vi "modifier main.vi"() -> ()   [LabVIEW 2013, in "vi mod UI.lvlib"]
doc: "This is the main VI for the configuration editor."
uses:
  vi mod UI.lvlib
  Controls/StateCluster.ctl
  <vilib>/NI/Configuration Framework/Repository/NISE_CEF_Repository.lvclass
  <vilib>/NI/Configuration Framework/Node/NodeRef.ctl
  <vilib>/NI/Configuration Framework/Node/NISE_CEF_Node.lvclass
  <vilib>/NI/Configuration Framework/Node/UserEventRef.ctl
  <vilib>/NI/Configuration Framework/Controls/EventCluster.ctl
  Controls/AddMessage.ctl
  Controls/MoveMessage.ctl
  modification container/modification container.lvclass
  collection/VI modification collection.lvclass
  <vilib>/NI/AMC/Read Termination Message.vi
  <vilib>/NI/AMC/Create Single Message.vi
  <vilib>/NI/AMC/Update Message Routing Info.vi
  <vilib>/NI/AMC/Send Message.vi
  <vilib>/NI/AMC/Globals.vi
  <vilib>/NI/AMC/AMC.lvlib
  <vilib>/NI/Configuration Framework/NISE_CEF_TreeControl.lvlib
panel:
  in  "stop":bool
  in  "View":string(tree)
  # "VI Modifier"
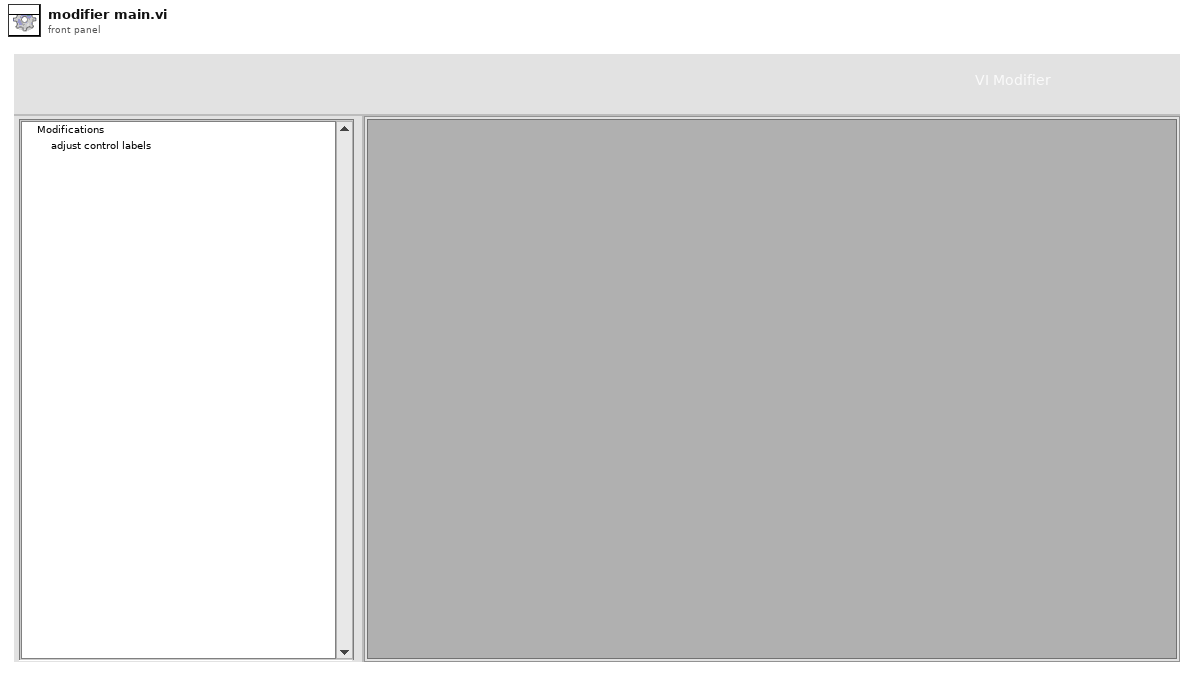
[diagram p1: front panel]
types:
  T1 = typedef "vi mod UI.lvlib/StateCluster.ctl" = cluster{"repository":refnum<class "NISE_CEF_Repository.lvclass">, "root":T2, "unsaved changes":bool, "current path":path, "user event ref":T3, "classes path":path}
  T2 = typedef "NISE_CEF_Node.lvclass/NodeRef.ctl" = refnum<data-value>
  T3 = typedef "NISE_CEF_Node.lvclass/UserEventRef.ctl" = refnum<user-event>
  T4 = typedef "AMC.lvlib/Message Queue.ctl" = refnum<queue>
  T5 = typedef "vi mod UI.lvlib/AddMessage.ctl" = cluster{"node type":string, "to add to":string}
  T6 = typedef "vi mod UI.lvlib/MoveMessage.ctl" = cluster{"node ref":T2, "new parent":T2}
  T7 = typedef "LVPoint32TypeDef.ctl" = cluster{"Horizontal":i32, "Vertical":i32}
  T8 = cluster{"data name":string, "drag data":variant}[]
  T9 = typedef "NISE_CEF_Node.lvclass/NodeMenuOptions.ctl" = cluster{"removable":bool, "movable":bool, "duplicate":bool}
  T10 = typedef "NISE_CEF_TreeControl.lvlib/EventCluster.ctl" = cluster{"command":string, "data":string}
  T11 = typedef "vi mod UI.lvlib/FilePaths.ctl" = cluster{"classes":path}
  T12 = typedef "NISE_CEF_Node.lvclass/Summary.ctl" = cluster{"ID":string, "parent ID":string, "node type":string, "text":string, "additional text":string, "glyph":string, "depth":i32, "glyph overlay":string}
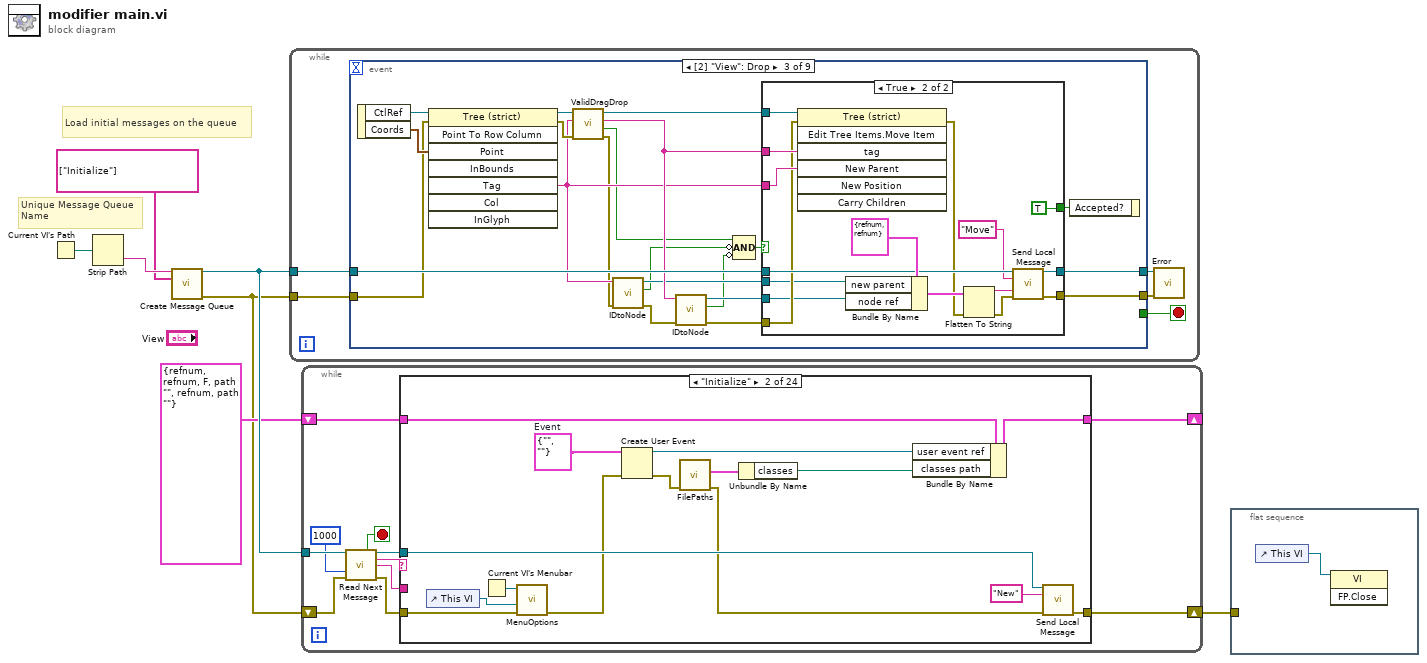
[diagram p0: block diagram]
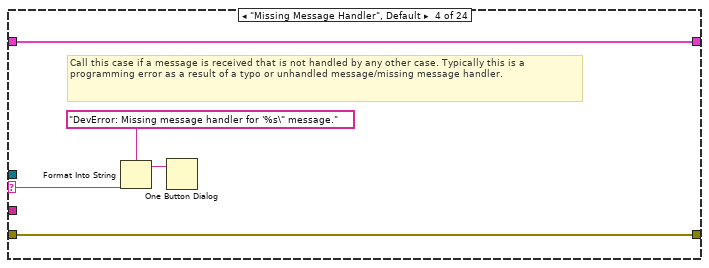
[diagram p4: hidden frame]
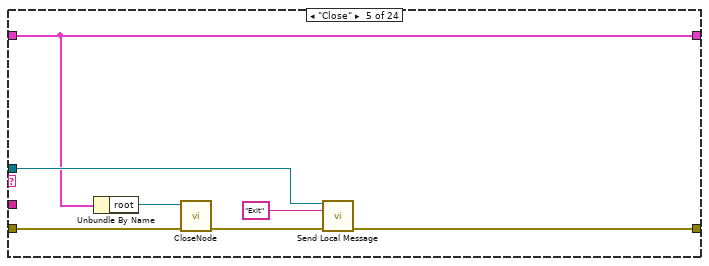
[diagram p5: hidden frame]
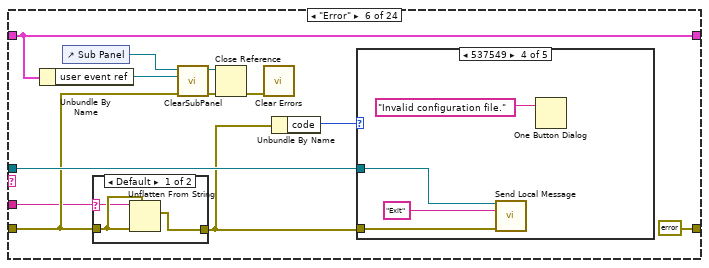
[diagram p6: hidden frame]
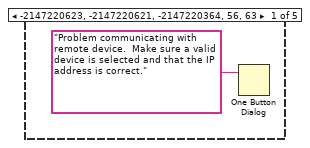
[diagram p8: hidden frame]
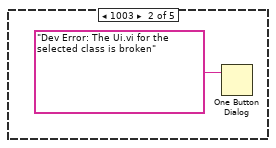
[diagram p9: hidden frame]
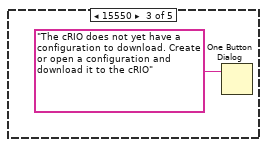
[diagram p10: hidden frame]
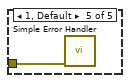
[diagram p11: hidden frame]
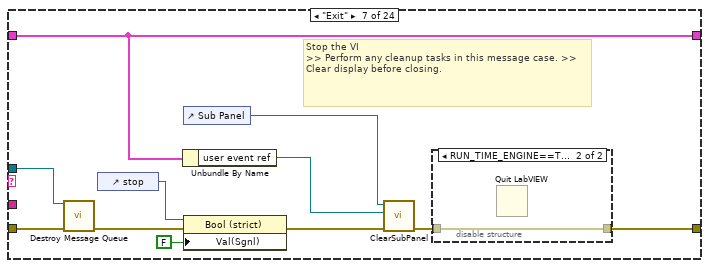
[diagram p12: hidden frame]
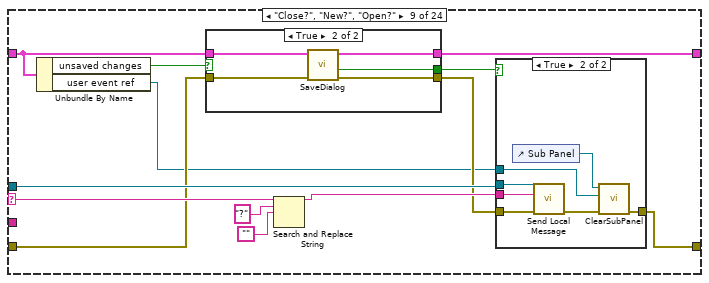
[diagram p15: hidden frame]
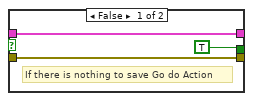
[diagram p16: hidden frame]
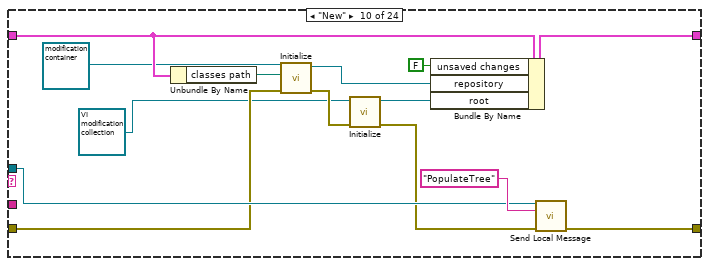
[diagram p18: hidden frame]
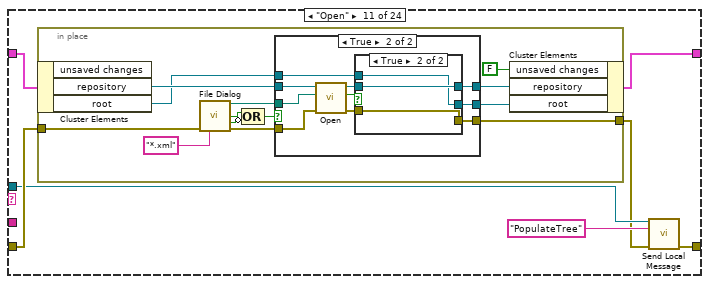
[diagram p19: hidden frame]
diagram:
  # "Unique Message Queue Name"
  # "Load initial messages on the queue"
  n1 = Current VI's Path() -> (path=w6:path)
  n2 = Strip Path(path=w6) -> (name=w7:string)  [unwired: 1 out]
  n3 = call <vilib>:"Create Message Queue.vi"("message queue name"=w7, "initial message names"=string[] ["Initialize"]) -> ("message queue out"=w4:T4, "error out"=w2:errorcluster)  [unwired: 12 in]
  n4 = while "User Interface Event Handler" {
    tunnel: w4 -> [w12]
    tunnel: w2 -> [w8]
    stop <- w11 stop-if-true
    n5 = event shown="[2] \"View\": Drop" {
      selector: _ -> [_ _ _ _ _ _ _ _ _]
      dyn-events: _ -> [_ _ _ _ _ _ _ _ _]
      timeout: _ -> [_ _ _ _ _ _ _ _ _]
      tunnel: w12 -> [w20 w44 w96 w124 w151 w155 w165 w171 w176]
      tunnel: [_ _ _ _ _ _ _ TRUE _] -> w11
      tunnel: [w20 w41 w94 w124 w148 w155 w163 w170 w175] -> w10
      tunnel: [w16 w40 w93 w120 w147 w152 w161 w168 w173] -> w9
      tunnel: w8 -> [w19 w39 w95 w123 w146 w154 w162 w169 w174]
      event "View": Shortcut Menu Activation? {
        n6 = event-data() -> ("CtlRef"=w26:refnum<vi>, "Coords"=w25:T7, "MenuRef"=w22:refnum<k9>)  [unwired: 1 in]
        n7 = invoke class="Tree (strict)" method="Point To Row Column"(reference=w26, error in=w19, "Point"=w25) -> (error out=w18:errorcluster, "Tag"=w24:string)  [unwired: 5 in, 6 out]
        n8 = call <vilib>:"IDtoNode.vi"("error in"=w18, "ID"=w24) -> ("error out"=w14:errorcluster, "invalid Id"=w21:bool, "node ref"=w23:T2)  [unwired: 7 in]
        n9 = case shown="False" w21 {
          tunnel: w23 -> [w31 _]
          tunnel: w22 -> [w30 _]
          tunnel: [w29 _] -> w17
          tunnel: [w28 _] -> w15
          tunnel: w14 -> [w27 w37]
          tunnel: [w27 w37] -> w13
          frame False {
            n10 = in-place {
              in-place-border: w30 -> [w34]
              in-place-border: [w32] -> w29
              n11 = in-place-dvr #1(w31) -> (w36:refnum<class "NISE_CEF_Node.lvclass">, w33:errorcluster)
              n12 = call-dynamic "ShortcutMenu.vi"("error in"=w33, "menu ref in"=w34, "node in"=w36) -> ("error out"=w32:errorcluster, "node out"=w35:refnum<class "NISE_CEF_Node.lvclass">)  [unwired: 6 in, 1 out]
              n13 = in-place-dvr #1(w35) -> (w28:errorcluster)  [unwired: 1 out]
            }
          }
          frame True {
          }
        }
        n14 = Merge Errors(w15, w17, w13) -> (w16:errorcluster)
        n15 = event-data() -> ()  [unwired: 2 in, 1 out]
      }
      event "View": Shortcut Menu Selection (User) {
        n16 = event-data() -> ("ItemPath"=w43:string, "CtlRef"=w47:refnum<vi>, "Coords"=w48:T7)  [unwired: 1 in]
        n17 = invoke class="Tree (strict)" method="Point To Row Column"(reference=w47, error in=w39, "Point"=w48) -> (error out=w38:errorcluster, "Tag"=w42:string)  [unwired: 5 in, 6 out]
        n18 = Match Pattern(string=w43, regular expression=":") -> (before substring=w46:string, after substring=w45:string)  [unwired: 1 in, 2 out]
        n19 = case shown="Default" w46 {
          selector: w46 -> [w50 _ _ _]
          tunnel: w45 -> [_ _ _ w75]
          tunnel: w44 -> [w57 w64 w70 w77]
          tunnel: w42 -> [w52 w62 w68 w76]
          tunnel: [w54 w61 w67 w73] -> w41
          tunnel: [w55 w60 w65 w71] -> w40
          tunnel: w38 -> [w56 w59 w66 w72]
          frame Default {
            n20 = Concatenate Strings(w50, ":" ("string"), w52) -> (w53:string)
            n21 = call <vilib>:"Send Local Message.vi"("message queue in"=w57, "message name"="CustomMenuAction" ("Message Name"), "message value"=w53, "error in"=w56) -> ("message queue out"=w54:T4, "error out"=w55:errorcluster)  [unwired: 9 in, 1 out]
          }
          frame "Remove" {
            n22 = call <vilib>:"Send Local Message.vi"("message queue in"=w64, "message name"="RemoveNode" ("Message Name"), "message value"=w62, "error in"=w59) -> ("message queue out"=w61:T4, "error out"=w60:errorcluster)  [unwired: 9 in, 1 out]
          }
          frame "Duplicate" {
            n23 = call <vilib>:"Send Local Message.vi"("message queue in"=w70, "message name"="Duplicate" ("Message Name"), "message value"=w68, "error in"=w66) -> ("message queue out"=w67:T4, "error out"=w65:errorcluster)  [unwired: 9 in, 1 out]
          }
          frame "Add" {
            n24 = Bundle By Name(cluster=T5 {"node type"="", "to add to"=""} ("input cluster"), "node type"=w75, "to add to"=w76) -> (w78:T5)
            n25 = Flatten To String(anything=w78) -> (data string=w79:string)  [unwired: 3 in, 2 out]
            n26 = call <vilib>:"Send Local Message.vi"("message queue in"=w77, "message name"="AddNode" ("Message Name"), "message value"=w79, "error in"=w72) -> ("message queue out"=w73:T4, "error out"=w71:errorcluster)  [unwired: 9 in, 1 out]
          }
        }
      }
      event "View": Drop {
        n27 = event-data() -> ("CtlRef"=w99:refnum<vi>, "Coords"=w98:T7)  [unwired: 1 in]
        n28 = invoke class="Tree (strict)" method="Point To Row Column"(reference=w99, error in=w95, "Point"=w98) -> (reference out=w97:refnum<vi>, error out=w92:errorcluster, "Tag"=w89:string)  [unwired: 5 in, 5 out]
        n29 = call <vilib>:"ValidDragDrop.vi"("error in"=w92, "drag over"=w89, "tree ref in"=w97) -> ("error out"=w84:errorcluster, "accepted"=w87:bool, "drag"=w91:string, "tree ref out"=w101:refnum<vi>)  [unwired: 5 in]
        n30 = call <vilib>:"IDtoNode.vi"("error in"=w84, "ID"=w89) -> ("error out"=w85:errorcluster, "invalid Id"=w82:bool, "node ref"=w88:T2)  [unwired: 7 in]
        n31 = call <vilib>:"IDtoNode.vi"("error in"=w85, "ID"=w91) -> ("error out"=w83:errorcluster, "invalid Id"=w81:bool, "node ref"=w90:T2)  [unwired: 7 in]
        n32 = Compound Arithmetic op=AND(w87, invert w82, invert w81) -> (w86:bool)
        n33 = case shown="True" w86 {
          tunnel: w91 -> [_ w117]
          tunnel: w101 -> [_ w119]
          tunnel: [_ TRUE] -> w100
          tunnel: w89 -> [_ w115]
          tunnel: w96 -> [w103 w114]
          tunnel: [w103 w110] -> w94
          tunnel: [w102 w109] -> w93
          tunnel: w90 -> [_ w105]
          tunnel: w88 -> [_ w104]
          tunnel: w83 -> [w102 w106]
          frame False {
          }
          frame True {
            n34 = invoke class="Tree (strict)" method="Edit Tree Items.Move Item"(reference=w119, error in=w106, "tag"=w117, "New Parent"=w115) -> (error out=w107:errorcluster)  [unwired: 3 in, 6 out]
            n35 = Bundle By Name(cluster=T6 {"node ref"=refnum, "new parent"=refnum} ("Cluster"), "new parent"=w104, "node ref"=w105) -> (w113:T6)
            n36 = Flatten To String(anything=w113, error in (no error)=w107) -> (data string=w112:string, error out=w108:errorcluster)  [unwired: 2 in, 1 out]
            n37 = call <vilib>:"Send Local Message.vi"("message queue in"=w114, "message name"="Move", "message value"=w112, "error in"=w108) -> ("message queue out"=w110:T4, "error out"=w109:errorcluster)  [unwired: 9 in, 1 out]
          }
        }
        n38 = event-data("Accepted?"=w100) -> ()  [unwired: 1 in, 1 out]
      }
      event "View": Drag Starting? {
        n39 = event-data() -> ("Data"=w130:T8, "CtlRef"=w132:refnum<vi>, "Coords"=w131:T7)  [unwired: 1 in]
        n40 = invoke class="Tree (strict)" method="Point To Row Column"(reference=w132, error in=w123, "Point"=w131) -> (error out=w122:errorcluster, "Tag"=w129:string)  [unwired: 5 in, 6 out]
        n41 = call <vilib>:"IDtoNode.vi"("error in"=w122, "ID"=w129) -> ("error out"=w121:errorcluster, "invalid Id"=w128:bool, "node ref"=w127:T2)  [unwired: 7 in]
        n42 = case shown="False" w128 {
          tunnel: w127 -> [w138 _]
          tunnel: [w135 TRUE ("Removable")] -> w125
          tunnel: w121 -> [w134 w144]
          tunnel: [w133 w144] -> w120
          frame False {
            n43 = in-place {
              in-place-border: [w141] -> w137
              in-place-border: w134 -> [w140]
              in-place-border: [w139] -> w133
              n44 = in-place-dvr #2(w138) -> (w143:refnum<class "NISE_CEF_Node.lvclass">)  [unwired: 1 out]
              n45 = call-dynamic "EditOptions.vi"("error in"=w140, "node in"=w143) -> ("error out"=w139:errorcluster, "edit options"=w141:T9, "node out"=w142:refnum<class "NISE_CEF_Node.lvclass">)  [unwired: 6 in, 1 out]
              n46 = in-place-dvr #2(w142) -> ()  [unwired: 2 out]
            }
            n47 = Unbundle By Name(w137) -> ("movable"=w136:bool)
            n48 = Not(x=w136) -> (.not. x?=w135:bool)
          }
          frame True {
          }
        }
        n49 = event-data("Data"=w130, "Drag Mode"=enum32{"copy or move", "copy only", "move only"}."move only", "Discard?"=w125) -> ()  [unwired: 1 in, 1 out]
      }
      event "View": Value Change {
        n50 = event-data() -> ("NewVal"=w149:string)  [unwired: 1 in]
        n51 = call <vilib>:"Send Local Message.vi"("message queue in"=w151, "message name"="ActivateNode" ("Message Name"), "message value"=w149, "error in"=w146) -> ("message queue out"=w148:T4, "error out"=w147:errorcluster)  [unwired: 9 in, 1 out]
      }
      event "View": event type 3.0.xa000003a {
        n52 = event-data() -> ("CtlRef"=w160:refnum<vi>, "Coords"=w157:T7)  [unwired: 1 in]
        n53 = invoke class="Tree (strict)" method="Point To Row Column"(reference=w160, error in=w154, "Point"=w157) -> (reference out=w159:refnum<vi>, error out=w153:errorcluster, "Tag"=w158:string)  [unwired: 5 in, 5 out]
        n54 = call <vilib>:"ValidDragDrop.vi"("error in"=w153, "drag over"=w158, "tree ref in"=w159) -> ("error out"=w152:errorcluster, "accepted"=w156:bool)  [unwired: 5 in, 2 out]
        n55 = event-data("Accepted?"=w156) -> ()  [unwired: 1 in, 1 out]
      }
      event Panel Close? {
        # "Intercepts the upper right close panel operation to allow a smooth shutdown as opposed to immediately killing the app."
        n56 = event-data() -> ()  [unwired: 1 in, 1 out]
        n57 = call <vilib>:"Send Local Message.vi"("message queue in"=w165, "message name"="Close?", "error in"=w162) -> ("message queue out"=w163:T4, "error out"=w161:errorcluster)  [unwired: 10 in, 1 out]
        n58 = event-data("Discard?"=TRUE) -> ()  [unwired: 1 in, 1 out]
      }
      event "stop": Value Change {
        n59 = event-data() -> ()  [unwired: 1 in, 1 out]
        n60 = call <vilib>:"Send Local Message.vi"("message queue in"=w171, "message name"="Close", "error in"=w169) -> ("message queue out"=w170:T4, "error out"=w168:errorcluster)  [unwired: 10 in, 1 out]
      }
      event Menu Selection (User) {
        # "#USERCFG It is needed to add a Case for Every item on the menu"
        n61 = event-data() -> ("ItemPath"=w177:string)  [unwired: 1 in]
        n62 = case shown="Default" w177 {
          tunnel: w176 -> [w179 w185 w190 w195 w200 w205 w214]
          tunnel: [w179 w181 w186 w191 w196 w201 w211] -> w175
          tunnel: w174 -> [w178 w183 w188 w193 w198 w203 w210]
          tunnel: [w178 w182 w187 w192 w197 w202 w208] -> w173
          frame Default {
            n63 = One Button Dialog(message="Unknown Menu Option") -> ()  [unwired: 1 in, 1 out]
          }
          frame "_File:_New" {
            n64 = call <vilib>:"Send Local Message.vi"("message queue in"=w185, "message name"="New?" ("Message Name"), "error in"=w183) -> ("message queue out"=w181:T4, "error out"=w182:errorcluster)  [unwired: 10 in, 1 out]
          }
          frame "_File:_Open" {
            n65 = call <vilib>:"Send Local Message.vi"("message queue in"=w190, "message name"="Open?" ("Message Name"), "error in"=w188) -> ("message queue out"=w186:T4, "error out"=w187:errorcluster)  [unwired: 10 in, 1 out]
          }
          frame "_File:_Save" {
            n66 = call <vilib>:"Send Local Message.vi"("message queue in"=w195, "message name"="Save" ("Message Name"), "error in"=w193) -> ("message queue out"=w191:T4, "error out"=w192:errorcluster)  [unwired: 10 in, 1 out]
          }
          frame "_File:Save As..." {
            n67 = call <vilib>:"Send Local Message.vi"("message queue in"=w200, "message name"="SaveAs" ("Message Name"), "error in"=w198) -> ("message queue out"=w196:T4, "error out"=w197:errorcluster)  [unwired: 10 in, 1 out]
          }
          frame "_File:_Exit" {
            n68 = call <vilib>:"Send Local Message.vi"("message queue in"=w205, "message name"="Close?" ("Message Name"), "error in"=w203) -> ("message queue out"=w201:T4, "error out"=w202:errorcluster)  [unwired: 10 in, 1 out]
          }
          frame "_Tools:Multiple Parameter Editor" {
            n69 = call <vilib>:"Send Local Message.vi"("message queue in"=w214, "message name"="CleansubPanel", "error in"=w210) -> ("message queue out"=w213:T4, "error out"=w209:errorcluster)  [unwired: 10 in, 1 out]
            n70 = call <vilib>:"Send Local Message.vi"("message queue in"=w213, "message name"="Custom View" ("Message Name"), "message value"="Multiple Variable Editor" ("Message Name"), "error in"=w209) -> ("message queue out"=w211:T4, "error out"=w208:errorcluster)  [unwired: 9 in, 1 out]
          }
        }
      }
    }
    n71 = call "Error.vi"("error in (no error)"=w9, "message queue in"=w10) -> ()  [unwired: 9 in, 1 out]
  }
  n72 = while "Message Processor" {
    shift-right: [w221] -> w1
    shift-left: w2 -> [w220]
    tunnel: w4 -> [w219]
    shift-right: [w217] -> _
    shift-left: T1 {"repository"=refnum, "root"=refnum, "unsaved changes"=FALSE, "current path"=path "", "user event ref"=refnum, "classes path"=path ""} -> [w216]
    stop <- w225 stop-if-true
    n73 = call <vilib>:"Read Next Message.vi"("message queue in"=w219, "timeout (1 ms)"=1000, "error in"=w220) -> ("exit process?"=w225:bool, "message queue out"=w215:T4, "message name"=w224:string, "message value"=w223:string, "error out"=w222:errorcluster)  [unwired: 5 in, 3 out]
    n74 = case shown="\"Initialize\"" w224 {
      selector: w224 -> [_ _ _ w246 _ _ _ _ w304 _ _ _ _ _ _ _ _ w487 _ _ _ _ _ _]
      tunnel: w223 -> [_ _ _ _ _ w257 _ _ _ _ _ _ _ w416 _ w455 w468 w485 w516 w539 _ _ w575 w597]
      tunnel: w222 -> [w227 w242 w244 w249 w251 w260 w291 w295 w297 w327 w343 w382 w408 w423 w436 w444 w467 w490 w518 w538 w555 w565 w574 w595]
      tunnel: [w227 w238 w244 w249 w255 errorcluster {"status"=FALSE, "code"=0, "source"=""} ("error out") w284 w295 w308 w337 w339 w386 w410 w420 w436 w447 w471 w493 w522 w535 w549 w560 w571 w590] -> w221
      tunnel: [w226 w233 w243 w245 w253 w265 w283 w294 w299 w335 w344 w389 w409 w417 w435 w438 w465 w494 w520 w533 w559 w564 w569 w586] -> w217
      tunnel: w216 -> [w226 w234 w243 w245 w253 w265 w283 w294 w300 w331 w345 w384 w407 w418 w435 w442 w472 w494 w521 w540 w559 w564 w569 w598]
      tunnel: w215 -> [_ w237 _ _ w254 w268 w290 _ w307 w336 w341 w385 _ w419 _ _ _ w488 _ _ _ _ w570 w589]
      frame "------------Generic Operations------------" {
        # "Dummy case to add a seperation in the Case Structure menu"
      }
      frame "Initialize" {
        w229 = T10 {"command"="", "data"=""}  # Event
        n75 = control-ref of="This VI"() -> (w241:refnum<vi>)
        n76 = Current VI's Menubar() -> (w240:refnum<k9>)
        n77 = call "MenuOptions.vi"("error in"=w242, "VI ref"=w241, "menu ref in"=w240) -> ("error out"=w232:errorcluster)  [unwired: 7 in, 1 out]
        n78 = Create User Event(user event datatype=w229, error in=w232) -> (user event=w228:refnum<user-event>, error out=w231:errorcluster)
        n79 = call "FilePaths.vi"("error in"=w231) -> ("error out"=w236:errorcluster, "paths"=w235:T11)  [unwired: 9 in]
        n80 = Unbundle By Name(w235) -> ("classes"=w230:path)
        n81 = Bundle By Name(cluster=w234, "user event ref"=w228, "classes path"=w230) -> (w233:T1)
        n82 = call <vilib>:"Send Local Message.vi"("message queue in"=w237, "message name"="New" ("Message Name"), "error in"=w236) -> ("error out"=w238:errorcluster)  [unwired: 10 in, 2 out]
      }
      frame "", "Idle" {
      }
      frame "Missing Message Handler", Default {
        # "Call this case if a message is received that is not handled by any other case. Typically this is a programming error as a result of a typo or unhandled message/missing message handler."
        n83 = Format Into String(format string="DevError: Missing message handler for '%s\" message." ("message"), w246) -> (resulting string=w248:string)  [unwired: 2 in, 1 out]
        n84 = One Button Dialog(message=w248) -> ()  [unwired: 2 out]
      }
      frame "Close" {
        n85 = Unbundle By Name(w253) -> ("root"=w252:T2)
        n86 = call <vilib>:"CloseNode.vi"("error in"=w251, "node ref"=w252) -> ("error out"=w250:errorcluster)  [unwired: 9 in]
        n87 = call <vilib>:"Send Local Message.vi"("message queue in"=w254, "message name"="Exit", "error in"=w250) -> ("error out"=w255:errorcluster)  [unwired: 10 in, 2 out]
      }
      frame "Error" {
        n88 = Unbundle By Name(w265) -> ("user event ref"=w263:T3)
        n89 = control-ref of="Sub Panel"() -> (w264:refnum<vi>)
        n90 = case shown="Default" w257 {
          selector: w257 -> [w270 _]
          tunnel: w260 -> [w271 w272]
          tunnel: [w269 w272] -> w259
          frame Default {
            n91 = Unflatten From String(type=w271, binary string=w270, error in (no error)=w271) -> (value=w269:errorcluster)  [unwired: 2 in, 2 out]
          }
          frame "" {
          }
        }
        n92 = call <vilib>:"ClearSubPanel.vi"("error in"=w260, "user event ref"=w263, "sub panel ref in"=w264) -> ("error out"=w262:errorcluster, "sub panel ref out"=w261:refnum<vi>)  [unwired: 7 in]
        n93 = Close Reference(reference=w261, error in (no error)=w262) -> (error out=w258:errorcluster)
        n94 = call <vilib>:"Clear Errors.vi"("error in (no error)"=w258) -> ()  [unwired: 6 in, 1 out]
        n95 = Unbundle By Name(w259) -> ("code"=w266:i32)
        n96 = case shown="537549" w266 {
          tunnel: w268 -> [_ _ _ w278 _]
          tunnel: w259 -> [_ _ _ w277 w280]
          frame -2147220623, -2147220621, -2147220364, 56, 63 {
            n97 = One Button Dialog(message="Problem communicating with remote device.  Make sure a valid device is selected and that the IP address is correct.") -> ()  [unwired: 1 in, 1 out]
          }
          frame 1003 {
            n98 = One Button Dialog(message="Dev Error: The Ui.vi for the selected class is broken") -> ()  [unwired: 1 in, 1 out]
          }
          frame 15550 {
            n99 = One Button Dialog(message="The cRIO does not yet have a configuration to download. Create or open a configuration and download it to the cRIO") -> ()  [unwired: 1 in, 1 out]
          }
          frame 537549 {
            n100 = call <vilib>:"Send Local Message.vi"("message queue in"=w278, "message name"="Exit", "error in"=w277) -> ()  [unwired: 10 in, 3 out]
            n101 = One Button Dialog(message="Invalid configuration file.") -> ()  [unwired: 1 in, 1 out]
          }
          frame 1, Default {
            n102 = call <vilib>:"Simple Error Handler.vi"("error in (no error)"=w280) -> ()  [unwired: 1 in, 8 out]
          }
        }
      }
      frame "Exit" {
        # "Stop the VI                                                                             >> Perform any cleanup tasks in this message case. >> Clear display before closing."
        n103 = call <vilib>:"Destroy Message Queue.vi"("message queue in"=w290, "error in"=w291) -> ("error out"=w288:errorcluster)  [unwired: 11 in, 2 out]
        n104 = control-ref of="stop"() -> (w281:refnum<vi>)
        n105 = Unbundle By Name(w283) -> ("user event ref"=w282:T3)
        n106 = control-ref of="Sub Panel"() -> (w287:refnum<vi>)
        n107 = property class="Bool (strict)"(reference=w281, error in=w288, "Val(Sgnl)"=FALSE ("Exit")) -> (error out=w286:errorcluster)  [unwired: 1 out]
        n108 = call <vilib>:"ClearSubPanel.vi"("error in"=w286, "user event ref"=w282, "sub panel ref in"=w287) -> ("error out"=w285:errorcluster)  [unwired: 7 in, 1 out]
        n109 = disable-structure shown="RUN_TIME_ENGINE==True" {
          disable-tunnel: [w292 w293] -> w284
          disable-tunnel: w285 -> [w292 w293]
          frame condition #0 (active) {
          }
          frame condition #1 {
            n110 = Quit LabVIEW() -> ()  [unwired: 1 in]
          }
        }
      }
      frame "------------Menu Operations--------------" {
        # "Dummy case to add a seperation in the Case Structure menu"
      }
      frame "Close?", "New?", "Open?" {
        n111 = Unbundle By Name(w300) -> ("unsaved changes"=w302:bool, "user event ref"=w296:T3)
        n112 = case shown="True" w302 {
          tunnel: [TRUE ("SaveFlag") w316] -> w301
          tunnel: w300 -> [w310 w315]
          tunnel: [w310 w314] -> w299
          tunnel: w297 -> [w309 w313]
          tunnel: [w309 w312] -> w298
          frame False {
            # "If there is nothing to save Go do Action"
          }
          frame True {
            n113 = call "SaveDialog.vi"("error in"=w313, "state in"=w315) -> ("error out"=w312:errorcluster, "new"=w316:bool, "state out"=w314:T1)  [unwired: 7 in]
          }
        }
        n114 = Search and Replace String(input string=w304, search string="?", replace string="") -> (result string=w303:string)  [unwired: 5 in, 3 out]
        n115 = case shown="True" w301 {
          tunnel: w298 -> [w317 w324]
          tunnel: [w317 w320] -> w308
          tunnel: w307 -> [_ w323]
          tunnel: w303 -> [_ w322]
          tunnel: w296 -> [_ w319]
          frame False {
          }
          frame True {
            n116 = control-ref of="Sub Panel"() -> (w318:refnum<vi>)
            n117 = call <vilib>:"Send Local Message.vi"("message queue in"=w323, "message name"=w322, "error in"=w324) -> ("error out"=w321:errorcluster)  [unwired: 10 in, 2 out]
            n118 = call <vilib>:"ClearSubPanel.vi"("error in"=w321, "user event ref"=w319, "sub panel ref in"=w318) -> ("error out"=w320:errorcluster)  [unwired: 7 in, 1 out]
          }
        }
      }
      frame "New" {
        n119 = Unbundle By Name(w331) -> ("classes path"=w330:path)
        n120 = call-dynamic "Initialize.vi"("error in"=w327, "path"=w330, "repository in"=refnum<class "modification container.lvclass"> refnum ("modification container.lvclass")) -> ("error out"=w329:errorcluster, "repository out"=w332:refnum<class "modification container.lvclass">)  [unwired: 7 in]
        n121 = call-dynamic "Initialize.vi"("error in"=w329, "node in"=refnum<class "VI modification collection.lvclass"> refnum ("VI modification collection.lvclass")) -> ("error out"=w328:errorcluster, "data value reference"=w333:T2)  [unwired: 7 in, 1 out]
        n122 = Bundle By Name(cluster=w331, "unsaved changes"=FALSE ("SaveFlag"), "repository"=w332, "root"=w333) -> (w335:T1)
        n123 = call <vilib>:"Send Local Message.vi"("message queue in"=w336, "message name"="PopulateTree", "error in"=w328) -> ("error out"=w337:errorcluster)  [unwired: 10 in, 2 out]
      }
      frame "Open" {
        n124 = in-place {
          in-place-border: w343 -> [w351]
          in-place-border: [w355] -> w340
          n125 = in-place-cluster #3(w345) -> ("repository"=w358:refnum<class "NISE_CEF_Repository.lvclass">, "root"=w349:T2)  [unwired: 1 out]
          n126 = call "File Dialog"("error in"=w351, "pattern (all files)"="*.xml") -> ("selected path"=w352:path, "exists"=w348:bool, "cancelled"=w347:bool, "error out"=w350:errorcluster)  [unwired: 10 in]
          n127 = Compound Arithmetic op=OR(w348, invert w347) -> (w346:bool)
          n128 = case shown="True" w346 {
            tunnel: w358 -> [w359 w371]
            tunnel: [w359 w369] -> w356
            tunnel: [w360 w367] -> w355
            tunnel: [w361 w366] -> w354
            tunnel: w352 -> [_ w364]
            tunnel: w350 -> [w360 w363]
            tunnel: w349 -> [w361 w362]
            frame False {
            }
            frame True {
              n129 = call-dynamic "Open.vi"("error in"=w363, "file path"=w364, "repository in"=w371) -> ("error out"=w368:errorcluster, "invalid?"=w365:bool, "repository out"=w370:refnum<class "NISE_CEF_Repository.lvclass">)  [unwired: 6 in]
              n130 = case shown="True" w365 {
                tunnel: w370 -> [w376 w379]
                tunnel: [w375 w379] -> w369
                tunnel: w368 -> [w374 w378]
                tunnel: [w373 w378] -> w367
                tunnel: [w372 w377] -> w366
                tunnel: w362 -> [_ w377]
                frame False {
                  n131 = call-dynamic "WriteTree.vi"("error in"=w374, "repository in"=w376) -> ("error out"=w373:errorcluster, "root"=w372:T2, "repository out"=w375:refnum<class "NISE_CEF_Repository.lvclass">)  [unwired: 7 in]
                }
                frame True {
                }
              }
            }
          }
          n132 = in-place-cluster #3("unsaved changes"=FALSE ("SaveFlag"), "repository"=w356, "root"=w354) -> (w344:T1)
        }
        n133 = call <vilib>:"Send Local Message.vi"("message queue in"=w341, "message name"="PopulateTree", "error in"=w340) -> ("error out"=w339:errorcluster)  [unwired: 10 in, 2 out]
      }
      frame "Save" {
        n134 = in-place {
          in-place-border: w382 -> [w393]
          in-place-border: [w392] -> w381
          in-place-border: [w390] -> w380
          n135 = in-place-cluster #4(w384) -> ("current path"=w391:path, "root"=w394:T2, "repository"=w396:refnum<class "NISE_CEF_Repository.lvclass">)
          n136 = Empty String/Path?(string/path=w391) -> (empty?=w390:bool)
          n137 = call-dynamic "ReadTree.vi"("error in"=w393, "root"=w394, "repository in"=w396) -> ("error out"=w392:errorcluster, "repository out"=w395:refnum<class "NISE_CEF_Repository.lvclass">)  [unwired: 7 in]
          n138 = in-place-cluster #4("current path"=w391, "root"=w394, "repository"=w395) -> (w383:T1)
        }
        n139 = case shown="True" w380 {
          tunnel: w383 -> [w400 w402]
          tunnel: [w399 w401] -> w389
          tunnel: [w398 w403] -> w387
          tunnel: w381 -> [w397 w404]
          frame False {
            n140 = call "Save.vi"("error in"=w397, "state in"=w400) -> ("error out"=w398:errorcluster, "state out"=w399:T1)  [unwired: 8 in]
          }
          frame True {
            # "Empty path use Dialog"
            n141 = call "SaveAs.vi"("error in"=w404, "state in"=w402) -> ("error out"=w403:errorcluster, "state out"=w401:T1)  [unwired: 7 in, 1 out]
          }
        }
        n142 = call <vilib>:"Send Local Message.vi"("message queue in"=w385, "message name"="PopulateTree", "error in"=w387) -> ("error out"=w386:errorcluster)  [unwired: 10 in, 2 out]
      }
      frame "SaveAs" {
        n143 = in-place {
          in-place-border: w408 -> [w412]
          in-place-border: [w411] -> w406
          n144 = in-place-cluster #5(w407) -> ("root"=w413:T2, "repository"=w415:refnum<class "NISE_CEF_Repository.lvclass">)
          n145 = call-dynamic "ReadTree.vi"("error in"=w412, "root"=w413, "repository in"=w415) -> ("error out"=w411:errorcluster, "repository out"=w414:refnum<class "NISE_CEF_Repository.lvclass">)  [unwired: 7 in]
          n146 = in-place-cluster #5("root"=w413, "repository"=w414) -> (w405:T1)
        }
        n147 = call "SaveAs.vi"("error in"=w406, "state in"=w405) -> ("error out"=w410:errorcluster, "state out"=w409:T1)  [unwired: 7 in, 1 out]
      }
      frame "Custom View" {
        n148 = in-place {
          in-place-border: w423 -> [w434]
          in-place-border: [w433] -> w421
          in-place-border: w416 -> [w424]
          n149 = in-place-cluster #6(w418) -> ("repository"=w428:refnum<class "NISE_CEF_Repository.lvclass">, "root"=w427:T2)
          n150 = call-dynamic "ReadTree.vi"("error in"=w434, "root"=w427, "repository in"=w428) -> ("error out"=w431:errorcluster, "repository out"=w430:refnum<class "NISE_CEF_Repository.lvclass">)  [unwired: 7 in]
          n151 = call-dynamic "CustomView.vi"("error in"=w431, "view name"=w424, "repository in"=w430) -> ("error out"=w432:errorcluster, "repository out"=w429:refnum<class "NISE_CEF_Repository.lvclass">)  [unwired: 7 in]
          n152 = call-dynamic "WriteTree.vi"("error in"=w432, "repository in"=w429) -> ("error out"=w433:errorcluster, "root"=w425:T2, "repository out"=w426:refnum<class "NISE_CEF_Repository.lvclass">)  [unwired: 7 in]
          n153 = in-place-cluster #6("repository"=w426, "root"=w425) -> (w417:T1)
        }
        n154 = call <vilib>:"Send Local Message.vi"("message queue in"=w419, "message name"="PopulateTree", "error in"=w421) -> ("error out"=w420:errorcluster)  [unwired: 10 in, 2 out]
      }
      frame "-------TreeControl Operations-----------" {
        # "Dummy case to add a seperation in the Case Structure menu"
      }
      frame "AddNode" {
        n155 = Unflatten From String(type=T5 {"node type"="", "to add to"=""} ("input cluster"), binary string=w455) -> (value=w453:T5)  [unwired: 3 in, 2 out]
        n156 = Unbundle By Name(w453) -> ("to add to"=w450:string, "node type"=w440:string)
        n157 = in-place {
          in-place-border: w444 -> [w461]
          in-place-border: [w460] -> w443
          in-place-border: w440 -> [w459]
          in-place-border: [w458] -> w439
          n158 = in-place-cluster #7(w442) -> ("repository"=w463:refnum<class "NISE_CEF_Repository.lvclass">)
          n159 = call-dynamic "GetClassPath.vi"("error in"=w461, "class name"=w459, "Repository in"=w463) -> ("error out"=w460:errorcluster, "class path"=w458:path, "Repository out"=w462:refnum<class "NISE_CEF_Repository.lvclass">)  [unwired: 6 in]
          n160 = in-place-cluster #7("repository"=w462) -> (w441:T1)
        }
        n161 = control-ref of="View"() -> (w445:refnum<vi>)
        n162 = call <vilib>:"Get LV Class Default Value.vi"("error in (no error)"=w443, "class path"=w439) -> ("error out"=w456:errorcluster, "object"=w457:refnum<class>)  [unwired: 8 in]
        n163 = To More Specific Class(target class=refnum<class "NISE_CEF_Node.lvclass"> refnum ("Node.lvclass"), reference=w457, error in=w456) -> (specific class reference=w452:refnum<class "NISE_CEF_Node.lvclass">, error out=w449:errorcluster)
        n164 = Bundle By Name(cluster=w441, "unsaved changes"=TRUE) -> (w438:T1)
        n165 = call <vilib>:"AddNode.vi"("error in"=w449, "node in"=w452, "parent node ID"=w450) -> ("error out"=w448:errorcluster, "summary"=w446:T12[])  [unwired: 7 in]
        n166 = call <vilib>:"PopulateTreeSumary.vi"("error in"=w448, "array"=w446, "tree ref in"=w445) -> ("error out"=w447:errorcluster)  [unwired: 8 in]
      }
      frame "Duplicate" {
        n167 = call <vilib>:"IDtoNode.vi"("error in"=w467, "ID"=w468) -> ("error out"=w469:errorcluster, "invalid Id"=w466:bool, "node ref"=w470:T2)  [unwired: 7 in]
        n168 = case shown="False" w466 {
          tunnel: [w481 w482] -> w471
          tunnel: w470 -> [w479 _]
          tunnel: w469 -> [w476 w482]
          frame False {
            n169 = call <vilib>:"DuplicateNode.vi"("same parent?"=TRUE ("s"), "error in"=w476, "node ref in"=w479) -> ("error out"=w477:errorcluster, "new node ref"=w478:T2)  [unwired: 7 in]
            n170 = call <vilib>:"Summary.vi"("error in"=w477, "node self ref"=w478) -> ("error out"=w474:errorcluster, "summary"=w473:T12[])  [unwired: 8 in]
            n171 = control-ref of="View"() -> (w480:refnum<vi>)
            n172 = call <vilib>:"PopulateTreeSumary.vi"("error in"=w474, "array"=w473, "tree ref in"=w480) -> ("error out"=w481:errorcluster)  [unwired: 8 in]
          }
          frame True {
          }
        }
        n173 = Bundle By Name(cluster=w472, "unsaved changes"=TRUE) -> (w465:T1)
      }
      frame "CustomMenuAction" {
        n174 = Match Pattern(string=w485, regular expression=":") -> (before substring=w484:string, after substring=w483:string)  [unwired: 1 in, 2 out]
        n175 = call <vilib>:"IDtoNode.vi"("error in"=w490, "ID"=w483) -> ("error out"=w491:errorcluster, "invalid Id"=w489:bool, "node ref"=w492:T2)  [unwired: 7 in]
        n176 = case shown="False" w489 {
          tunnel: [w497 w513] -> w493
          tunnel: w492 -> [w501 _]
          tunnel: w491 -> [w498 w513]
          tunnel: w488 -> [w500 _]
          tunnel: w487 -> [_ _]
          tunnel: w484 -> [w495 _]
          frame False {
            n177 = control-ref of="View"() -> (w499:refnum<vi>)
            n178 = in-place {
              in-place-border: w500 -> [w511]
              in-place-border: w499 -> [w509]
              in-place-border: w498 -> [w508]
              in-place-border: [w507] -> w497
              in-place-border: [w506] -> w496
              in-place-border: w495 -> [w505]
              n179 = in-place-dvr #8(w501) -> (w512:refnum<class "NISE_CEF_Node.lvclass">)  [unwired: 1 out]
              n180 = call-dynamic "MenuHandler.vi"("tree control"=w509, "main message queue"=w511, "error in"=w508, "menu string"=w505, "NISE_CEF_Node in"=w512) -> ("error out"=w507:errorcluster, "Unhandled"=w506:bool, "NISE_CEF_Node out"=w510:refnum<class "NISE_CEF_Node.lvclass">)  [unwired: 3 in, 1 out]
              n181 = in-place-dvr #8(w510) -> ()  [unwired: 2 out]
            }
            n182 = case shown="True" w496 {
              tunnel: w495 -> [_ w502]
              frame False {
              }
              frame True {
                # "Generates Error"
                n183 = Concatenate Strings("Unknown item command:  " ("message"), w502) -> (w504:string)
                n184 = One Button Dialog(message=w504) -> ()  [unwired: 1 in, 1 out]
              }
            }
          }
          frame True {
          }
        }
      }
      frame "RefreshNode" {
        # "Refreshes the node in the Tree               Sets the save flag to true                       This case can be called from the UIs of the nodes"
        n185 = call <vilib>:"IDtoNode.vi"("error in"=w518, "ID"=w516) -> ("error out"=w517:errorcluster, "invalid Id"=w514:bool, "node ref"=w515:T2)  [unwired: 7 in]
        n186 = case shown="True" w514 {
          tunnel: [w529 w531] -> w522
          tunnel: w517 -> [w524 w531]
          tunnel: w515 -> [w523 _]
          frame False {
            n187 = call <vilib>:"Summary.vi"("error in"=w524, "node self ref"=w523) -> ("error out"=w526:errorcluster, "summary"=w525:T12[])  [unwired: 8 in]
            n188 = control-ref of="View"() -> (w527:refnum<vi>)
            n189 = call <vilib>:"RefreshSubTree.vi"("error in"=w526, "node information"=w525, "tree ref in"=w527) -> ("error out"=w530:errorcluster, "tree ref out"=w528:refnum<vi>)  [unwired: 7 in]
            n190 = Close Reference(reference=w528, error in (no error)=w530) -> (error out=w529:errorcluster)
          }
          frame True {
          }
        }
        n191 = Bundle By Name(cluster=w521, "unsaved changes"=TRUE ("SaveFlag")) -> (w520:T1)
      }
      frame "RemoveNode" {
        n192 = call <vilib>:"IDtoNode.vi"("error in"=w538, "ID"=w539) -> ("error out"=w537:errorcluster, "invalid Id"=w534:bool, "node ref"=w536:T2)  [unwired: 7 in]
        n193 = case shown="False" w534 {
          tunnel: w537 -> [w546 w547]
          tunnel: w536 -> [w545 _]
          tunnel: [w541 w547] -> w535
          frame False {
            n194 = call <vilib>:"RemoveNode.vi"("error in"=w546, "node"=w545) -> ("error out"=w542:errorcluster, "node ID"=w544:string)  [unwired: 8 in]
            n195 = control-ref of="View"() -> (w543:refnum<vi>)
            n196 = call <vilib>:"ClearTreeNode.vi"("error in"=w542, "tag"=w544, "tree reference"=w543) -> ("error out"=w541:errorcluster)  [unwired: 8 in]
          }
          frame True {
          }
        }
        n197 = Bundle By Name(cluster=w540, "unsaved changes"=TRUE) -> (w533:T1)
      }
      frame "PopulateTree" {
        n198 = Unbundle By Name(w559) -> ("user event ref"=w548:T3, "root"=w553:T2)
        n199 = call <vilib>:"Summary.vi"("error in"=w555, "depth"=0 ("Depth"), "node self ref"=w553) -> ("error out"=w554:errorcluster, "summary"=w558:T12[])  [unwired: 7 in]
        n200 = control-ref of="This VI"() -> (w556:refnum<vi>)
        n201 = control-ref of="View"() -> (w557:refnum<vi>)
        n202 = call <vilib>:"RefreshEntireTree.vi"("calling VI in"=w556, "error in"=w554, "array"=w558, "tree ref in"=w557) -> ("error out"=w550:errorcluster)  [unwired: 7 in]
        n203 = control-ref of="Sub Panel"() -> (w551:refnum<vi>)
        n204 = call <vilib>:"ClearSubPanel.vi"("error in"=w550, "user event ref"=w548, "sub panel ref in"=w551) -> ("error out"=w549:errorcluster)  [unwired: 7 in, 1 out]
      }
      frame "CleansubPanel" {
        n205 = Unbundle By Name(w564) -> ("user event ref"=w563:T3)
        n206 = control-ref of="Sub Panel"() -> (w566:refnum<vi>)
        n207 = call <vilib>:"ClearSubPanel.vi"("error in"=w565, "user event ref"=w563, "sub panel ref in"=w566) -> ("error out"=w562:errorcluster, "sub panel ref out"=w561:refnum<vi>)  [unwired: 7 in]
        n208 = Close Reference(reference=w561, error in (no error)=w562) -> (error out=w560:errorcluster)
      }
      frame "ActivateNode" {
        n209 = Unbundle By Name(w569) -> ("user event ref"=w568:T3)
        n210 = call <vilib>:"IDtoNode.vi"("error in"=w574, "ID"=w575) -> ("error out"=w567:errorcluster, "invalid Id"=w573:bool, "node ref"=w572:T2)  [unwired: 7 in]
        n211 = case shown="False" w573 {
          tunnel: w572 -> [w582 _]
          tunnel: [w583 w584] -> w571
          tunnel: w567 -> [w580 w584]
          tunnel: w570 -> [w577 _]
          tunnel: w568 -> [w578 _]
          frame False {
            n212 = control-ref of="Sub Panel"() -> (w579:refnum<vi>)
            n213 = call <vilib>:"ClearSubPanel.vi"("error in"=w580, "user event ref"=w578, "sub panel ref in"=w579) -> ("error out"=w581:errorcluster, "sub panel ref out"=w576:refnum<vi>)  [unwired: 7 in]
            n214 = call <vilib>:"LoadNodeUI.vi"("user event out"=w578, "error in"=w581, "sub panel ref in"=w576, "main queue"=w577, "node"=w582) -> ("error out"=w583:errorcluster)  [unwired: 6 in]
          }
          frame True {
          }
        }
      }
      frame "Move" {
        n215 = Unflatten From String(type=T6 {"node ref"=refnum, "new parent"=refnum} ("Cluster"), binary string=w597, error in (no error)=w595) -> (value=w594:T6, error out=w593:errorcluster)  [unwired: 2 in, 1 out]
        n216 = Unbundle By Name(w594) -> ("node ref"=w588:T2, "new parent"=w587:T2)
        n217 = call <vilib>:"MoveNode.vi"("error in"=w593, "new parent"=w587, "node"=w588) -> ("error out"=w591:errorcluster)  [unwired: 8 in]
        n218 = call <vilib>:"Send Local Message.vi"("message queue in"=w589, "message name"="PopulateTree", "error in"=w591) -> ("error out"=w590:errorcluster)  [unwired: 10 in, 2 out]
        n219 = Bundle By Name(cluster=w598, "unsaved changes"=TRUE) -> (w586:T1)
      }
    }
  }
  n220 = flat-sequence {
    tunnel: w1 -> [_]
    frame #0 {
      n221 = control-ref of="This VI"() -> (w599:refnum<vi>)
      n222 = invoke class="VI" method="FP.Close"(reference=w599) -> ()  [unwired: 2 in, 3 out]
    }
  }
